vi "Actor Core.vi"(8 "error in":errorcluster, 11 "He Line in":refnum<class "He Line.lvclass">) -> (0 "error out":errorcluster, 3 "Actor out":refnum<class "Actor.lvclass">)   [LabVIEW 2015, in "cRIO-Carbondioxide.lvlib" / "CO2-Actor.lvlib" / "He Line.lvclass"]
doc: "(<B>Filename</B>: Actor Framework.lvlib:Actor.lvclass:Actor Core.vi)\n\nReceives messages to the actor, reacts to them, and initiates any error handling that may shut the actor down.\n\nDescendant classes may override this VI to append parallel tasks for the actor to complete while it handles messages. Overrides use the Call Parent Method node."
uses:
  He Line.lvclass
  <vilib>/ActorFramework/Actor/Actor.lvclass
  Valve/Valve.lvclass
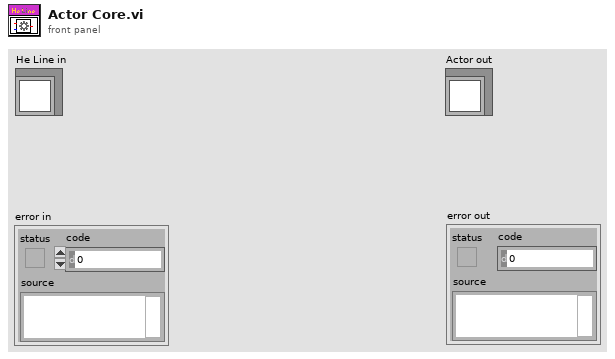
[diagram p1: front panel]
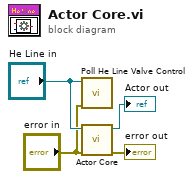
[diagram p0: block diagram]
diagram:
  n1 = call "Poll He Line Valve Control.vi"("error in (no error)"="error in", "He Line in"="He Line in") -> ()  [unwired: 10 in]
  n2 = call-parent "Actor Core.vi"("error in"="error in", "CO2 Actor in"="He Line in") -> ("error out"=→"error out":errorcluster, "Actor out"=→"Actor out":refnum<class "Actor.lvclass">)  [unwired: 8 in]
